vi "Read permissions.vi"(8 "error in (no error)":errorcluster, 11 "Shared Memory in":refnum<class "Shared Memory.lvclass">) -> (0 "error out":errorcluster, 2 "permissions":T1, 3 "Shared Memory out":refnum<class "Shared Memory.lvclass">)   [LabVIEW 2013, in "Linux RT IPC.lvlib" / "Shared Memory.lvlib" / "Shared Memory.lvclass"]
uses:
  Shared Memory.lvclass
  Shared Memory.lvclass/Shared Memory.ctl
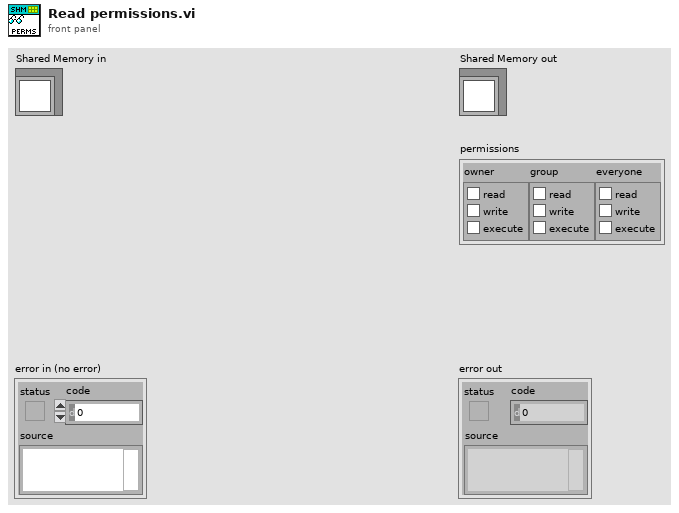
[diagram p1: front panel]
types:
  T1 = cluster{"owner":cluster{"read":bool, "write":bool, "execute":bool}, "group":cluster{"read":bool, "write":bool, "execute":bool}, "everyone":cluster{"read":bool, "write":bool, "execute":bool}}
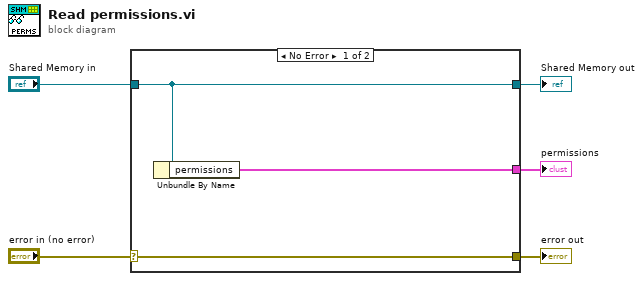
[diagram p0: block diagram]
diagram:
  n1 = case shown="No Error" "error in (no error)" {
    selector: "error in (no error)" -> [w8 w9]
    tunnel: [w8 w9] -> w4
    tunnel: [w7 w10] -> w2
    tunnel: "Shared Memory in" -> [w7 w10]
    tunnel: [w6 _] -> w1
    frame No Error {
      n2 = Unbundle By Name(w7) -> ("permissions"=w6:T1)
    }
    frame Error {
    }
  }
  "error out" <- w4
  "Shared Memory out" <- w2
  "permissions" <- w1
